vi "Seating plan.vi"(8 "error in (no error)":errorcluster, 11 "Table in":refnum<class "Table.lvclass">) -> (0 "error out":errorcluster, 3 "Table out":refnum<class "Table.lvclass">)   [LabVIEW 2023, in "Table.lvlib" / "Table.lvclass"]
uses:
  Table.lvclass
  Table.lvclass/Table.ctl
  <vilib>/Utility/miscctls.llb/LVRectTypeDef.ctl
  Philosopher/Philosopher Messages/Take Your Seat Msg/Take Your Seat.lvclass/Take Your Seat.ctl
  <vilib>/ActorFramework/Message Enqueuer/Message Enqueuer.lvclass/Message Enqueuer.ctl
  <vilib>/ActorFramework/Message Enqueuer/Enqueue.vi
  Philosopher/Philosopher Messages/Take Your Seat Msg/Take Your Seat.lvclass
  C:/Program Files (x86)/National Instruments/LabVIEW 2023/vi.lib/ActorFramework/Message/Message.lvclass
  <vilib>/ActorFramework/Message Priority Queue/Priority Enqueue.vi
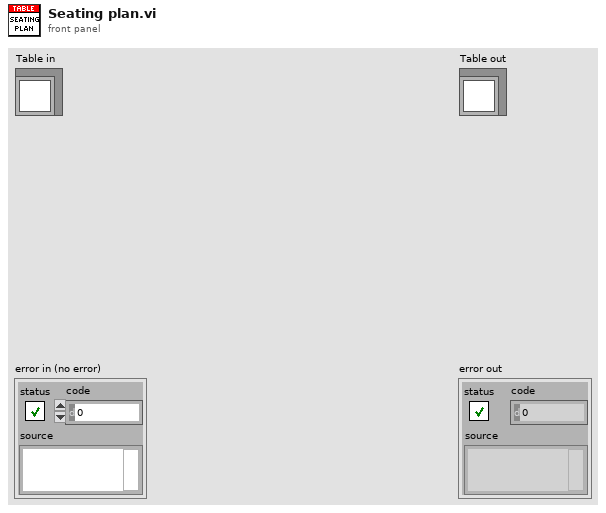
[diagram p1: front panel]
types:
  T1 = typedef "LVRectTypeDef.ctl" = cluster{"Left":i16, "Top":i16, "Right":i16, "Bottom":i16}
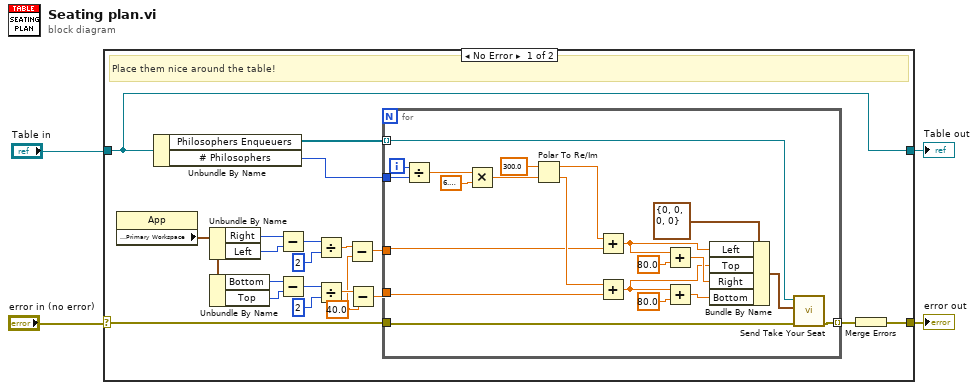
[diagram p0: block diagram]
diagram:
  n1 = case shown="No Error" "error in (no error)" {
    selector: "error in (no error)" -> [w21 w47]
    tunnel: [w20 w47] -> w3
    tunnel: [w24 w46] -> w1
    tunnel: "Table in" -> [w24 w46]
    frame No Error {
      w5 = 40.0 ("y")
      # "Place them nice around the table!"
      n2 = property class="App"() -> ("Display:Primary Workspace"=w14:T1)  [unwired: 2 in, 2 out]
      n3 = Unbundle By Name(w24) -> ("Philosophers Enqueuers"=w23:refnum<class "Message Enqueuer.lvclass">[], "# Philosophers"=w22:i32)
      n4 = Unbundle By Name(w14) -> ("Right"=w18:i16, "Left"=w17:i16)
      n5 = Unbundle By Name(w14) -> ("Bottom"=w11:i16, "Top"=w10:i16)
      n6 = Subtract(x=w18, y=w17) -> (x-y=w16:i16)
      n7 = Subtract(x=w11, y=w10) -> (x-y=w12:i16)
      n8 = Divide(x=w16, y=i16 2) -> (x/y=w8:dbl)
      n9 = Divide(x=w12, y=i16 2) -> (x/y=w7:dbl)
      n10 = Subtract(x=w8, y=w5) -> (x-y=w9:dbl)
      n11 = Subtract(x=w7, y=w5) -> (x-y=w6:dbl)
      n12 = for {
        tunnel: w23 -> [w29] mode=indexing
        tunnel: w22 -> [w31]
        tunnel: w21 -> [w27]
        tunnel: [w28] -> w19 mode=indexing
        tunnel: w6 -> [w26]
        tunnel: w9 -> [w25]
        i -> [w32]
        n13 = Divide(x=w32, y=w31) -> (x/y=w45:dbl)
        n14 = Multiply(x=w45, y=6.283185307179586) -> (x*y=w43:dbl)
        n15 = Polar To Re/Im(2:w43, 3:300.0 ("r")) -> (0:w40:dbl, 1:w41:dbl)
        n16 = Add(x=w41, y=w25) -> (x+y=w38:dbl)
        n17 = Add(x=w40, y=w26) -> (x+y=w35:dbl)
        n18 = Add(x=w38, y=80.0) -> (x+y=w36:dbl)
        n19 = Add(x=w35, y=80.0) -> (x+y=w34:dbl)
        n20 = Bundle By Name(cluster=T1 {"Left"=0, "Top"=0, "Right"=0, "Bottom"=0} ("Front Panel Window:Window Bounds"), "Left"=w38, "Top"=w35, "Right"=w36, "Bottom"=w34) -> (w30:T1)
        n21 = call "Send Take Your Seat.vi"("error in (no error)"=w27, "Front Panel Window:Panel Bounds"=w30, "Message Enqueuer"=w29) -> ("error out"=w28:errorcluster)  [unwired: 7 in, 1 out]
      }
      n22 = Merge Errors(w19) -> (w20:errorcluster)
    }
    frame Error {
    }
  }
  "error out" <- w3
  "Table out" <- w1
